vi "Get marker name.vi"() -> (1 "cancelled":bool, 3 "text":string)   [LabVIEW 2020, in "Graph Extensions.lvlib"]
uses:
  Graph Extensions.lvlib
  <vilib>/Utility/miscctls.llb/LVRectTypeDef.ctl
  <vilib>/Utility/inputDevices.llb/mouseAcquire.vi
panel:
  in  "Text":string
  in  "OK":bool
  in  "Cancel":bool
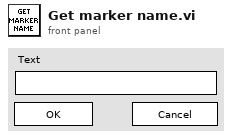
[diagram p1: front panel]
types:
  T1 = typedef "LVRectTypeDef.ctl" = cluster{"Left":i16, "Top":i16, "Right":i16, "Bottom":i16}
  T2 = cluster{"Horizontal":i32, "Vertical":i32, "Scrolling":i32}
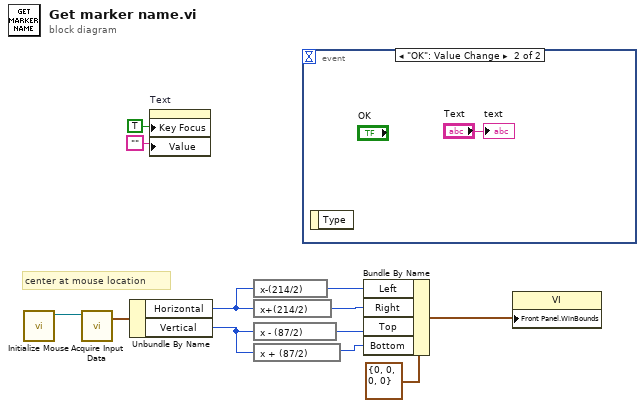
[diagram p0: block diagram]
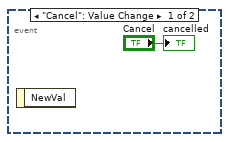
[diagram p2: hidden frame]
diagram:
  # "center at mouse location"
  n1 = call <vilib>:"Initialize Mouse.vi"() -> ("device ID"=w10:refnum<k1>)  [unwired: 10 in, 1 out]
  n2 = call-poly <vilib>:"Acquire Input Data.vi"("device ID"=w10) -> ("axis info"=w9:T2)  [unwired: 15 in, 3 out]
  n3 = Unbundle By Name(w9) -> ("Horizontal"=w2:i32, "Vertical"=w3:i32)
  n4 = property on="Text" class="Str"("Key Focus"=TRUE, "Value"="" ("Text")) -> ()  [unwired: 2 in, 2 out]
  n5 = expression code="x-(214/2)"(w2) -> (w6:i32)
  n6 = expression code="x+(214/2)"(w2) -> (w7:i32)
  n7 = expression code="x - (87/2)"(w3) -> (w5:i32)
  n8 = expression code="x + (87/2)"(w3) -> (w4:i32)
  n9 = event shown="[1] \"OK\": Value Change" {
    selector: _ -> [_ _]
    dyn-events: _ -> [_ _]
    timeout: _ -> [_ _]
    event "Cancel": Value Change {
      n10 = event-data() -> ()  [unwired: 1 in, 1 out]
      "cancelled" <- "Cancel"
    }
    event "OK": Value Change {
      n11 = event-data() -> ()  [unwired: 1 in, 1 out]
      "text" <- "Text"
    }
  }
  n12 = Bundle By Name(cluster=T1 {"Left"=0, "Top"=0, "Right"=0, "Bottom"=0} ("Front Panel Window:Window Bounds"), "Left"=w6, "Right"=w7, "Top"=w5, "Bottom"=w4) -> (w1:T1)
  n13 = property class="VI"("Front Panel.WinBounds"=w1) -> ()  [unwired: 2 in, 2 out]
